vi "RecordDataToEventProgressData.vi"(9 "RecordData":string[][](array[string]), 10 "inputEventProgressData":string[][](array[string])) -> (2 "outputEventProgressData":string[][](array[string]))   [LabVIEW 2020]
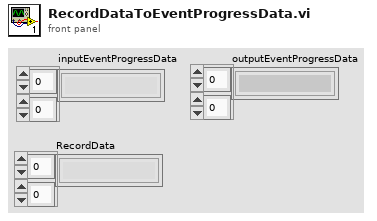
[diagram p1: front panel]
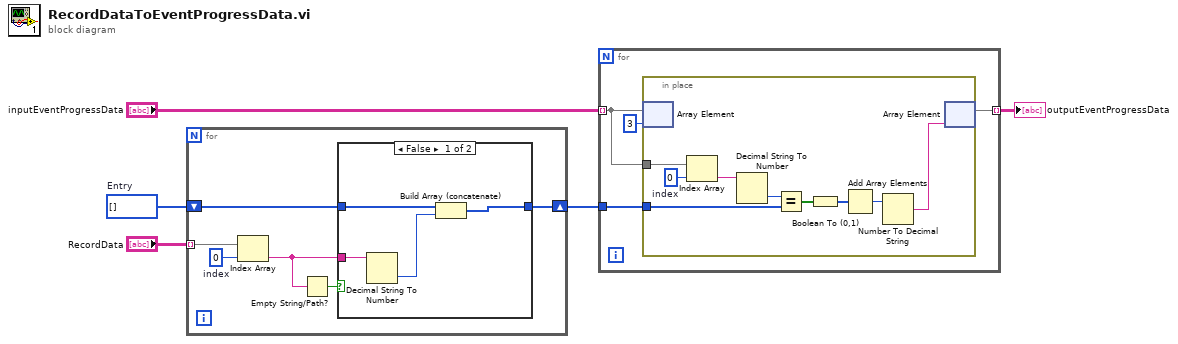
[diagram p0: block diagram]
diagram:
  w4 = i32[] []  # Entry
  n1 = for {
    tunnel: "RecordData" -> [w11] mode=indexing
    shift-right: [w6] -> w2
    shift-left: w4 -> [w7]
    w10 = 0  # index
    n2 = Index Array "Index Array"(array=w11, index=w10) -> (element=w8:string)
    n3 = Empty String/Path?(string/path=w8) -> (empty?=w9:bool)
    n4 = case shown="False" w9 {
      tunnel: w8 -> [w15 _]
      tunnel: w7 -> [w14 w16]
      tunnel: [w12 w16] -> w6
      frame False {
        n5 = Decimal String To Number(string=w15) -> (number=w13:i32)  [unwired: 2 in, 1 out]
        n6 = Build Array (concatenate) "Build Array"(w14, w13) -> (w12:i32[])
      }
      frame True {
      }
    }
  }
  n7 = for {
    tunnel: "inputEventProgressData" -> [w17] mode=indexing
    tunnel: w2 -> [w20]
    tunnel: [w19] -> w1 mode=indexing
    n8 = in-place {
      in-place-border: w20 -> [w28]
      in-place-border: w17 -> [w24]
      w21 = 0  # index
      n9 = in-place-array #1(w17, 3) -> ()  [unwired: 1 out]
      n10 = Index Array "Index Array"(array=w24, index=w21) -> (element=w23:string)
      n11 = Decimal String To Number(string=w23) -> (number=w29:i32)  [unwired: 2 in, 1 out]
      n12 = Equal?(x=w29, y=w28) -> (x = y?=w27:bool[])
      n13 = Boolean To (0,1)(Boolean=w27) -> (0, 1=w26:i16[])
      n14 = Add Array Elements(numeric array=w26) -> (sum=w25:i16)
      n15 = Number To Decimal String(number=w25) -> (decimal integer string=w22:string)  [unwired: 1 in]
      n16 = in-place-array #1(w22) -> (w19:string[])  [unwired: 1 out]
    }
  }
  "outputEventProgressData" <- w1
